vi "BRAM read write process.vi"(5 "debug ctr reset":bool, 6 "dram.reset":bool, 8 "dram mode":T3, 11 "DRAM resources":T1={"DRAM read data FIFO"="", "DRAM write data FIFO"="", "DRAM request FIFO"="", "DRAM U512 memo"=refnum, "DMA data loader"="custom data", "BRAM read data FIFO"="", "BRAM write data FIFO"="", "BRAM request FIFO"="", "BRAM U512 memo"=refnum}) -> (2 "BRAM debug ctr":T2, 3 "last written addr":u32)   [LabVIEW 2019, in "TX burst sequencer.lvlib"]
uses:
  TX burst sequencer.lvlib
  DRAM mode.ctl
  DRAM resources.ctl
  <instrlib>/_niInstr/Memory/v1/FPGA/DRAM U512/niInstr Memory DRAM U512 v1 FPGA.lvclass
  <instrlib>/_niInstr/Memory/v1/FPGA/BRAM U512/niInstr Memory BRAM U512 v1 FPGA.lvclass
  C:/Program Files/National Instruments/LabVIEW 2019/instr.lib/_niInstr/Memory/v1/FPGA/BRAM/niInstr Memory BRAM v1 FPGA.lvclass
  <instrlib>/_niInstr/Memory/v1/FPGA/Memory/Public/Read Request.ctl
  <instrlib>/_niInstr/Memory/v1/FPGA/Memory/Public/Write Data.ctl
  <vilib>/rvi/DataTransferAndStorage/Container/Common/niFpgaContainerExecOnDevCompGetState.vi
  <vilib>/rvi/Emulation/niFpgaEmulationIsFPGAContextNoSignature.vi
  <vilib>/rvi/Emulation/niFpgaSctlEmulationGetInTimedLoop.vi
  <vilib>/rvi/errors/niFpgaSetErrorForExecOnDevCompSimple.vi
  <vilib>/rvi/eio/common/nirviEmuReportErrorAndStop.vi
  <vilib>/rvi/DataTransferAndStorage/Container/Common/niFpgaContainerGetUniqueNameForEmu.vi
  <vilib>/rvi/FIFO/Fifo_Resource/nirvififoEmulationSetSize.vi
  <vilib>/rvi/FIFO/Fifo_Resource/nirviFifoEmulationQueueMgr.vi
  <instcachedir>/0/nirviFifoEmulationQueueMgr_E5CAEC123FF24DC58D834DCA3CDAA9B5.lvgen/nirviFifoEmulationQueueMgr_E5CAEC123FF24DC58D834DCA3CDAA9B5_017.vi
  <vilib>/rvi/FIFO/Fifo_Resource/nirvififoEmulationDetermineInputValidOut.vi
  <vilib>/rvi/FIFO/Fifo_Resource/nirvififoEmulationCreateLock.vi
  <vilib>/rvi/Emulation/niFpgaProcessEmulError.vi
  <vilib>/rvi/FIFO/Fifo_Resource/nirvififoEmulationObtainLock.vi
  <vilib>/rvi/FIFO/Fifo_Resource/nirvififoEmulationReleaseLock.vi
  <vilib>/rvi/occurrence/nirviWaitOnOccurrenceBase.vi
  <vilib>/rvi/errors/nirviReportUnexpectedCaseInternalError.vi
  <vilib>/rvi/errors/nirviReportUnexpectedCaseInternalError (U32).vi
  <vilib>/Utility/error.llb/Clear Errors.vi
  <vilib>/rvi/interface/RandomDataEmulation/niFpgaRandomDataHandleErrors.vi
  <instcachedir>/0/nirviFifoEmulationQueueMgr_E5CAEC123FF24DC58D834DCA3CDAA9B5.lvgen/nirviFifoEmulationQueueMgr_E5CAEC123FF24DC58D834DCA3CDAA9B5_003.vi
  <instrlib>/_niInstr/Basic Elements/v1/FPGA/Private/Count Up U32.vi
  <instcachedir>/0/nirviFifoEmulationQueueMgr_E5CAEC123FF24DC58D834DCA3CDAA9B5.lvgen/nirviFifoEmulationQueueMgr_E5CAEC123FF24DC58D834DCA3CDAA9B5_011.vi
  <vilib>/rvi/DataTransferAndStorage/Container/XNode/niFpgaContainer.xnode
  <vilib>/rvi/FIFO/Fifo_Resource/niFpgaFifoEmulationRefIn.vi
  <instrlib>/_niInstr/Memory/v1/FPGA/Memory/niInstr Memory v1 FPGA.lvclass
  <instrlib>/_niInstr/Basic Elements/v1/FPGA/niInstr Basic Elements v1 FPGA.lvlib
  <instrlib>/_niInstr/Memory/v1/FPGA/BRAM/niInstr Memory BRAM v1 FPGA.lvclass
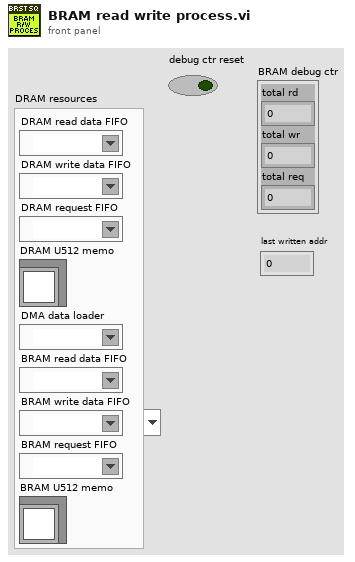
[diagram p1: front panel]
types:
  T1 = typedef "TX burst sequencer.lvlib/DRAM resources.ctl" = cluster{"DRAM read data FIFO":refnum<k21>, "DRAM write data FIFO":refnum<k21>, "DRAM request FIFO":refnum<k21>, "DRAM U512 memo":refnum<class "niInstr Memory DRAM U512 v1 FPGA.lvclass">, "DMA data loader":refnum<k21>, "BRAM read data FIFO":refnum<k21>, "BRAM write data FIFO":refnum<k21>, "BRAM request FIFO":refnum<k21>, "BRAM U512 memo":refnum<class "niInstr Memory BRAM U512 v1 FPGA.lvclass">}
  T2 = cluster{"total rd":u32, "total wr":u32, "total req":u32}
  T3 = typedef "TX burst sequencer.lvlib/DRAM mode.ctl" = enum16{"flush", "reset", "write", "read"}
  T4 = typedef "niInstr Memory v1 FPGA.lvclass/Write Data.ctl" = cluster{"address":u32, "data":bool[], "valid":bool}
  T5 = typedef "niInstr Memory v1 FPGA.lvclass/Read Request.ctl" = cluster{"address":u32, "valid":bool}
  T6 = typedef "niInstr Memory v1 FPGA.lvclass/Retrieve Data.ctl" = cluster{"data":bool[], "valid":bool}
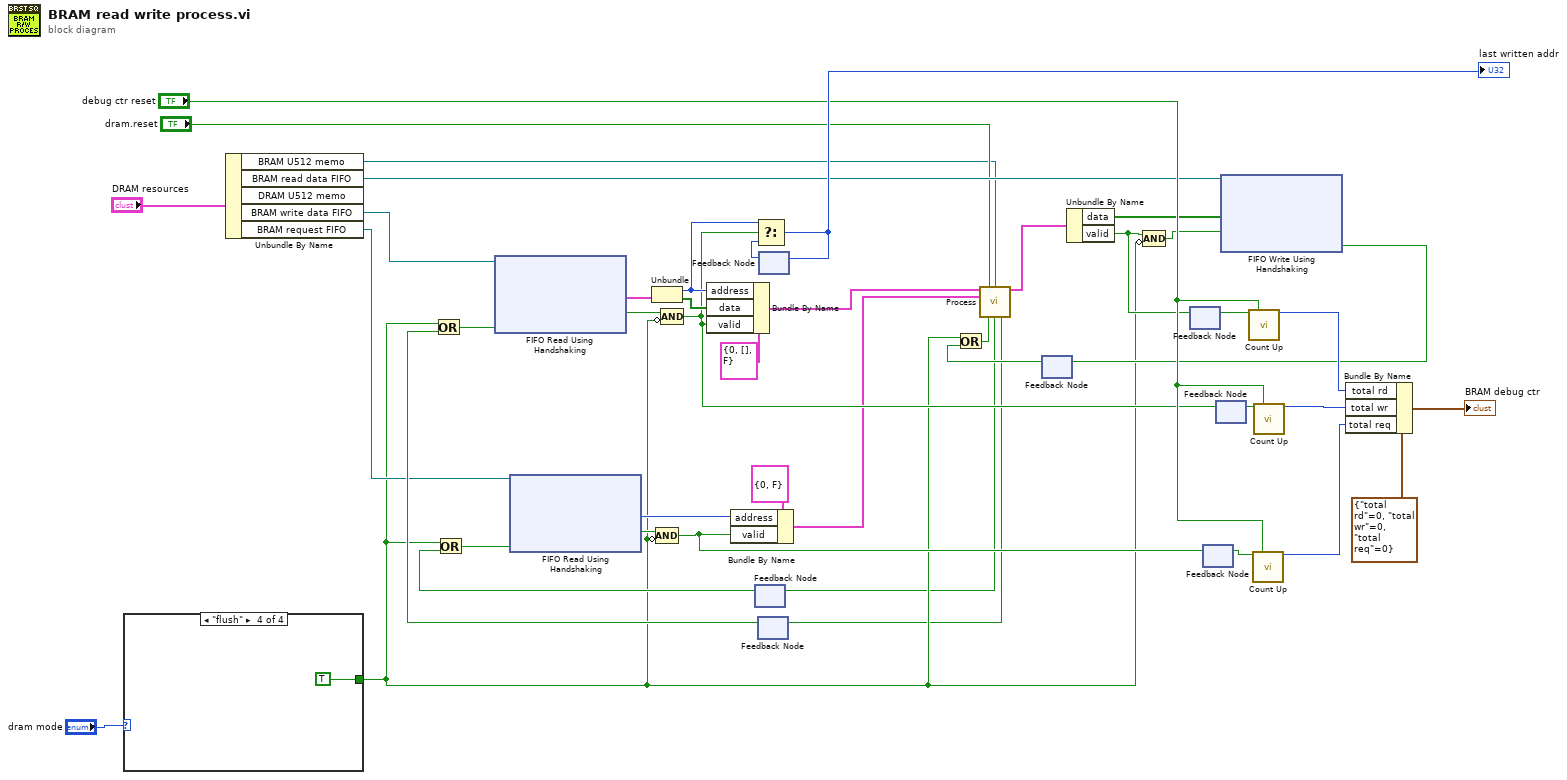
[diagram p0: block diagram]
diagram:
  n1 = case shown="\"flush\"" "dram mode" {
    tunnel: [_ _ _ TRUE] -> w11
    frame "read" {
    }
    frame Default {
    }
    frame "write" {
    }
    frame "flush" {
    }
  }
  n2 = Unbundle By Name("DRAM resources") -> ("BRAM U512 memo"=w1:refnum<class "niInstr Memory BRAM U512 v1 FPGA.lvclass">, "BRAM read data FIFO"=w21:refnum<k21>, "BRAM write data FIFO"=w20:refnum<k21>, "BRAM request FIFO"=w19:refnum<k21>)  [unwired: 1 out]
  n3 = feedback #1() -> (w30:bool)  [unwired: 1 in]
  n4 = Or(x=w11, y=w30) -> (x .or. y?=w18:bool)
  n5 = xnode ("FIFO Read Using Handshaking")("Ready for Output"=w18, "FIFO In"=w19) -> ("Element"=w29:u32, "Output Valid"=w34:bool)  [unwired: 1 out]
  n6 = Compound Arithmetic op=AND(w34, invert w11) -> (w16:bool)
  n7 = Bundle By Name(cluster=T5 {"address"=0, "valid"=FALSE} ("request data"), "address"=w29, "valid"=w16) -> (w7:T5)
  n8 = feedback #2() -> (w25:bool)  [unwired: 1 in]
  n9 = Or(x=w11, y=w25) -> (x .or. y?=w17:bool)
  n10 = xnode ("FIFO Read Using Handshaking")("Ready for Output"=w17, "FIFO In"=w20) -> ("Element"=w26:cluster{"addr":u32, "data":bool[]}, "Output Valid"=w15:bool)  [unwired: 1 out]
  n11 = Unbundle(w26) -> ("addr"=w36:u32, "data"=w27:bool[])
  n12 = Compound Arithmetic op=AND(w15, invert w11) -> (w14:bool)
  n13 = Bundle By Name(cluster=T4 {"address"=0, "data"=[], "valid"=FALSE} ("write"), "address"=w36, "data"=w27, "valid"=w14) -> (w8:T4)
  n14 = feedback #3() -> (w38:u32)  [unwired: 1 in]
  n15 = Select(t=w36, s=w14, f=w38) -> (s? t:f=w37:u32)
  "last written addr" <- w37
  n16 = feedback-in #3(w37) -> ()
  n17 = feedback #4() -> (w13:bool)  [unwired: 1 in]
  n18 = Or(x=w11, y=w13) -> (x .or. y?=w4:bool)
  n19 = call <instrlib>:"Process.vi"("write"=w8, "reset"="dram.reset", "memory"=w1, "request data"=w7, "ready for retrieve data (T)"=w4) -> ("retrieve data"=w6:T6, "ready for request data"=w3:bool, "ready for write"=w2:bool)  [unwired: 7 in, 1 out]
  n20 = feedback-in #1(w3) -> ()
  n21 = feedback-in #2(w2) -> ()
  n22 = Unbundle By Name(w6) -> ("data"=w23:bool[], "valid"=w12:bool)
  n23 = Compound Arithmetic op=AND(w12, invert w11) -> (w10:bool)
  n24 = feedback #5() -> (w32:bool)  [unwired: 1 in]
  n25 = feedback-in #5(w12) -> ()
  n26 = feedback #6() -> (w33:bool)  [unwired: 1 in]
  n27 = feedback-in #6(w16) -> ()
  n28 = feedback #7() -> (w31:bool)  [unwired: 1 in]
  n29 = feedback-in #7(w14) -> ()
  n30 = xnode ("FIFO Write Using Handshaking")("Element"=w23, "Input Valid"=w10, "FIFO In"=w21) -> ("Ready for Input"=w24:bool)  [unwired: 1 out]
  n31 = feedback-in #4(w24) -> ()
  n32 = call-poly <instrlib>:"Count Up.vi"("increment"=w32, "reset"="debug ctr reset") -> ("count out"=w40:u32)  [unwired: 13 in]
  n33 = call-poly <instrlib>:"Count Up.vi"("increment"=w33, "reset"="debug ctr reset") -> ("count out"=w42:u32)  [unwired: 13 in]
  n34 = call-poly <instrlib>:"Count Up.vi"("increment"=w31, "reset"="debug ctr reset") -> ("count out"=w41:u32)  [unwired: 13 in]
  n35 = Bundle By Name(cluster=T2 {"total rd"=0, "total wr"=0, "total req"=0} ("input cluster"), "total rd"=w40, "total wr"=w41, "total req"=w42) -> (→"BRAM debug ctr":T2)
